vi "Configure View Model.vi"(8 "error in (no error)":errorcluster, 10 "List Box View Model":refnum<class "Variant View Model.lvclass">, 11 "List Box View In":refnum<class "Variant View.lvclass">) -> (0 "error out":errorcluster, 3 "List Box View Out":refnum<class "Variant View.lvclass">)   [LabVIEW 2020, in "Variant View.lvclass"]
uses:
  Variant View.lvclass
  Variant View Model/Variant View Model.lvclass
  Variant View.lvclass/Variant View.ctl
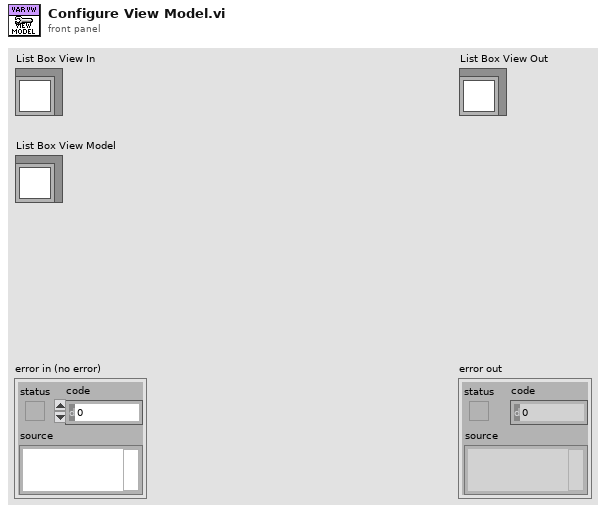
[diagram p1: front panel]
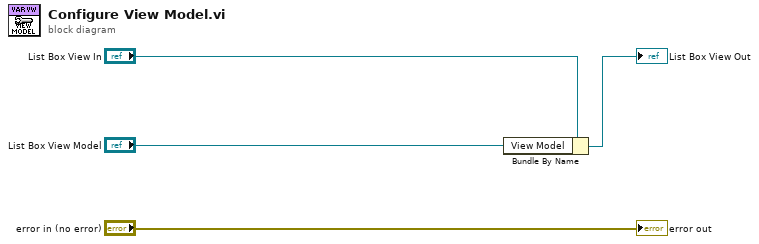
[diagram p0: block diagram]
diagram:
  n1 = Bundle By Name(cluster="List Box View In", "View Model"="List Box View Model") -> (→"List Box View Out":refnum<class "Variant View.lvclass">)
  "error out" <- "error in (no error)"
